vi "init temp chart property nodes.vi"(1 "Temperature History":refnum<vi>, 12 "range indicators":refnum<vi>[](array[refnum])) -> ()   [LabVIEW 2014]
doc: "This subvi inits various properties for the temperature controller\n\nMatt Strader\nPaul K Dixon\nPhysics 350\nPaul K Dixon"
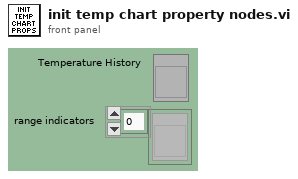
[diagram p1: front panel]
types:
  T1 = cluster{"Element Data":dbl, "Element Data":dbl, "Element Data":dbl, "Element Data":dbl, "Element Data":dbl, "Element Data":dbl, "Element Data":dbl}
  T2 = cluster{"Element Data":dbl, "Element Data":dbl, "Element Data":dbl, "Element Data":dbl, "Element Data":dbl, "Element Data":dbl, "Element Data":dbl}[]
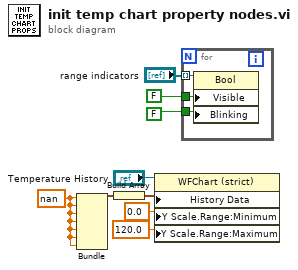
[diagram p0: block diagram]
diagram:
  w1 = nan ("Element Data")
  n1 = Bundle("Element Data"=w1, "Element Data"=w1, "Element Data"=w1, "Element Data"=w1, "Element Data"=w1, "Element Data"=w1, "Element Data"=w1) -> (w6:T1)  [unwired: 1 out]
  n2 = Build Array(w6) -> (w5:T2)
  n3 = property class="WFChart (strict)"(reference="Temperature History", "History Data"=w5, "Y Scale.Range:Minimum"=0.0, "Y Scale.Range:Maximum"=120.0) -> ()  [unwired: 1 in, 2 out]
  n4 = for {
    tunnel: "range indicators" -> [w12] mode=indexing
    tunnel: FALSE ("Visible") -> [w11]
    tunnel: FALSE ("Visible") -> [w10]
    n5 = property class="Bool"(reference=w12, "Visible"=w10, "Blinking"=w11) -> ()  [unwired: 1 in, 2 out]
  }
